vi "Calc Resistance (SubVI).vi"(7 "Configuration":enum16{"4-Band Code", "5-Band Code"}(ring), 8 "Band 3":u16, 9 "Band 2":u16, 10 "Band 1":u16) -> (1 "Format String":string, 2 "Resistance Value":i32, 3 "Visible":bool)   [LabVIEW 2012, in "Picture Box Tools.lvlib"]
uses:
  Picture Box Tools.lvlib
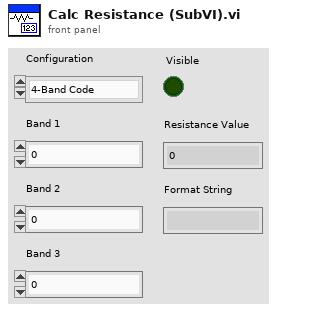
[diagram p1: front panel]
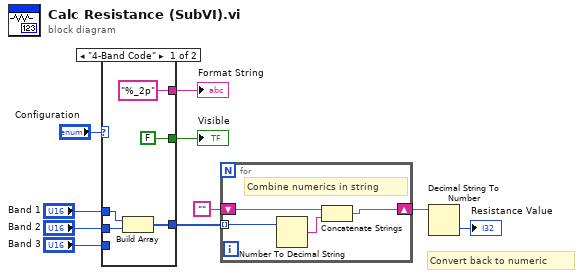
[diagram p0: block diagram]
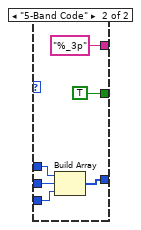
[diagram p2: hidden frame]
diagram:
  # "Convert back to numeric"
  n1 = case shown="\"4-Band Code\"" "Configuration" {
    tunnel: "Band 1" -> [w15 w20]
    tunnel: "Band 2" -> [w14 w21]
    tunnel: "Band 3" -> [_ w19]
    tunnel: [w13 w18] -> w5
    tunnel: [FALSE ("Visible") TRUE ("Visible")] -> w7
    tunnel: ["%_2p" ("format string") "%_3p" ("format string")] -> w10
    frame "4-Band Code" {
      n2 = Build Array(w15, w14) -> (w13:u16[])
    }
    frame "5-Band Code" {
      n3 = Build Array(w20, w21, w19) -> (w18:u16[])
    }
  }
  "Format String" <- w10
  "Visible" <- w7
  n4 = for {
    tunnel: w5 -> [w25] mode=indexing
    shift-right: [w23] -> w8
    shift-left: "" -> [w22]
    # "Combine numerics in string"
    n5 = Number To Decimal String(number=w25) -> (decimal integer string=w24:string)  [unwired: 1 in]
    n6 = Concatenate Strings(w22, w24) -> (w23:string)
  }
  n7 = Decimal String To Number(string=w8) -> (number=→"Resistance Value":i32)  [unwired: 2 in, 1 out]
